vi "Notify AE Monitoring.vi"(8 "error in (no error)":errorcluster, 11 "CS++DSCMonitor in":refnum<class "CS++DSCMonitor.lvclass">) -> (0 "error out":errorcluster, 3 "CS++DSCMonitor out":refnum<class "CS++DSCMonitor.lvclass">)   [LabVIEW 2015, in "CS++DSCMonitor.lvlib" / "CS++DSCMonitor.lvclass"]
doc: "Notify alarm and event monitoring."
uses:
  CS++DSCMonitor.lvclass
  CSPP_Core/Actors/CS++PVMonitor/CS++PVMonitor.lvclass/CS++PVMonitor.ctl
  CS++DSCMonitor.lvclass/CS++DSCMonitor.ctl
  <vilib>/ActorFramework/Message Enqueuer/Message Enqueuer.lvclass
  CSPP_Core/Actors/CS++PVMonitor Messages/CS++AEUpdate Msg/CS++AEUpdate Msg.lvclass
  CSPP_Core/Actors/CS++PVMonitor/CS++PVMonitor.lvclass
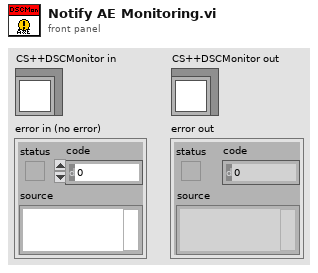
[diagram p1: front panel]
types:
  T1 = cluster{"PV URL":string, "Observers":cluster{"Enqueuer":refnum<class "Message Enqueuer.lvclass">, "CS++AEUpdate Msg":refnum<class "CS++AEUpdate Msg.lvclass">}[]}[]
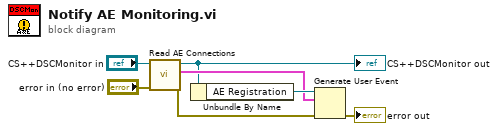
[diagram p0: block diagram]
diagram:
  n1 = call "Read AE Connections.vi"("error in (no error)"="error in (no error)", "CS++PVMonitor in"="CS++DSCMonitor in") -> ("error out"=w3:errorcluster, "AE Connections"=w4:T1, "CS++PVMonitor out"=w2:refnum<class "CS++DSCMonitor.lvclass">)  [unwired: 7 in]
  "CS++DSCMonitor out" <- w2
  n2 = Unbundle By Name(w2) -> ("AE Registration"=w7:refnum<user-event>)
  n3 = Generate User Event(user event=w7, event data cluster=w4, error in=w3) -> (error out=→"error out":errorcluster)  [unwired: 1 in, 1 out]
